vi "Set System Configuration.vi"(4 "error in (no error)":errorcluster, 6 "System Configuration":T1, 7 "VISA resource name":refnum<visa-resource-name>) -> (0 "error out":errorcluster, 3 "VISA resource name out":refnum<visa-resource-name>)   [LabVIEW 2014, in "Newport ESP301.lvlib"]
doc: "This command is used to configure system fault checking, event handling and general setup for all axes.\n<B>Note:</B> If bit-0 or both bits-1 and -2 are set to zero(0) then no action will be taken by the controller."
uses:
  Newport ESP301.lvlib
panel:
  # "queue purge on time expiration disabled"
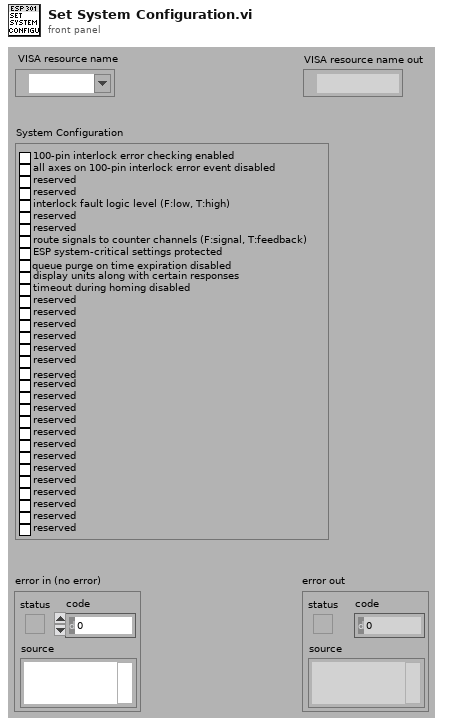
[diagram p1: front panel]
types:
  T1 = cluster{"100-pin interlock error checking enabled":bool, "all axes on 100-pin interlock error event disabled":bool, "reserved":bool, "reserved":bool, "interlock fault logic level (F:low, T:high)":bool, "reserved":bool, "reserved":bool, "route signals to counter channels (F:signal, T:feedback)":bool, "ESP system-critical settings protected":bool, bool, "display units along with certain responses ":bool, "timeout during homing disabled ":bool, "reserved ":bool, "reserved ":bool, "reserved ":bool, "reserved ":bool, "reserved ":bool, "reserved ":bool, "reserved ":bool, "reserved ":bool, "reserved ":bool, "reserved ":bool, "reserved ":bool, "reserved ":bool, "reserved ":bool, "reserved ":bool, "reserved ":bool, "reserved ":bool, "reserved ":bool, "reserved ":bool, "reserved ":bool, "reserved":bool}
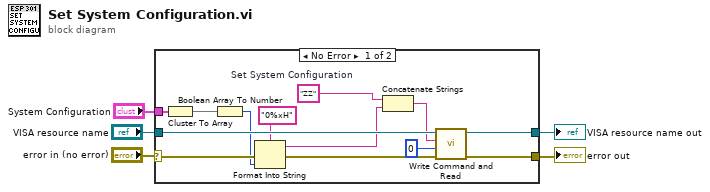
[diagram p0: block diagram]
diagram:
  n1 = case shown="No Error" "error in (no error)" {
    selector: "error in (no error)" -> [w11 w20]
    tunnel: [w17 w20] -> w5
    tunnel: "VISA resource name" -> [w18 w19]
    tunnel: [w16 w19] -> w4
    tunnel: "System Configuration" -> [w9 _]
    frame No Error {
      w15 = "ZZ"  # Set System Configuration
      n2 = Cluster To Array(cluster=w9) -> (array=w12:bool[])
      n3 = Boolean Array To Number(Boolean array=w12) -> (number=w8:u32)
      n4 = Format Into String(format string="0%xH" ("chaîne de format"), error in=w11, w8) -> (resulting string=w7:string, error out=w10:errorcluster)  [unwired: 1 in]
      n5 = Concatenate Strings(w15, w7) -> (w14:string)
      n6 = call "Write Command and Read.vi"("error in (no error)"=w10, "Bytes to read (100)"=u32 0, "Command"=w14, "VISA resource name"=w18) -> ("error out"=w17:errorcluster, "VISA resource name out"=w16:refnum<visa-resource-name>)  [unwired: 1 in, 3 out]
    }
    frame Error {
    }
  }
  "error out" <- w5
  "VISA resource name out" <- w4
